vi "MakeErrorObsolete.vi"(8 "ErrorIn":errorcluster caption="Error In(no Error)", 10 "ErrorCode":i32, 11 "ReferenceIn":refnum<class "ErrorDefinitionSQLite.lvclass"> caption="Reference In") -> (0 "ErrorOut":errorcluster caption="Error Out", 3 "ReferenceOut":refnum<class "ErrorDefinitionSQLite.lvclass"> caption="Reference Out")   [LabVIEW 2018, in "ErrorDefinitionSQLite.lvclass"]
uses:
  ErrorDefinitionSQLite.lvclass
  <vilib>/drjdpowell/SQLite Library/SQL Connection/Execute SQL.vi
  <vilib>/drjdpowell/SQLite Library/SQLite.lvlib
  <vilib>/drjdpowell/SQLite Library/SQL Connection/Connection.lvclass
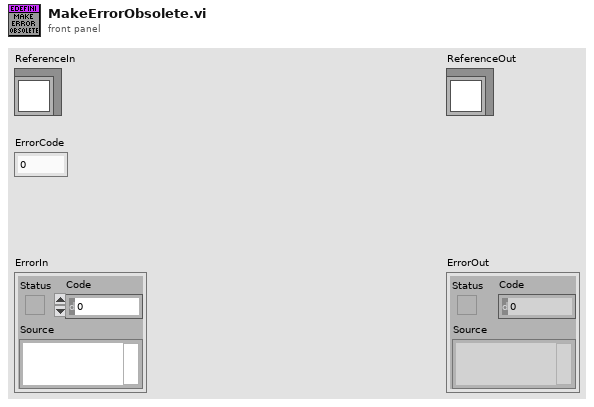
[diagram p1: front panel]
types:
  T1 = typedef "ErrorDefinitionSQLite.lvclass/ObjectAttributes.ctl" = cluster{"Path":path, "SQLiteRef":refnum<class "Connection.lvclass">, "EndOfRange":i32, "DefaultLibrarySize":i32, "StartOfRange":i32}
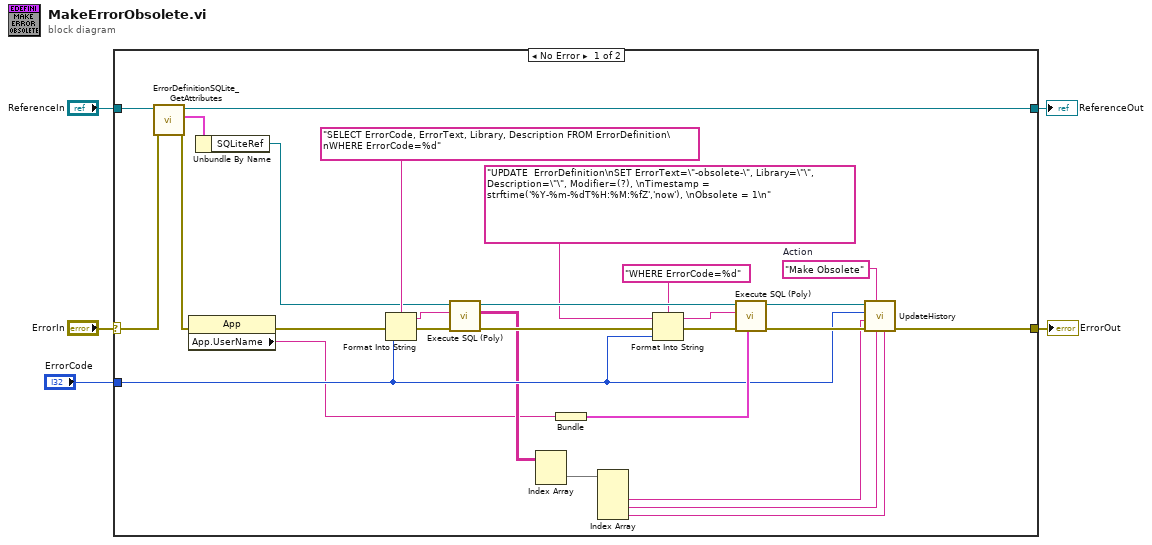
[diagram p0: block diagram]
diagram:
  n1 = case shown="No Error" "ErrorIn" {
    selector: "ErrorIn" -> [w33 w35]
    tunnel: [w6 w35] -> w4
    tunnel: [w31 w34] -> w2
    tunnel: "ReferenceIn" -> [w32 w34]
    tunnel: "ErrorCode" -> [w19 _]
    frame No Error {
      w26 = "Make Obsolete"  # Action
      n2 = call "ErrorDefinitionSQLite_GetAttributes.vi"("ErrorIn"=w33, "Reference in"=w32) -> ("ErrorOut"=w12:errorcluster, "Data"=w30:T1, "Reference out"=w31:refnum<class "ErrorDefinitionSQLite.lvclass">)  [unwired: 6 in, 1 out]
      n3 = property class="App"(error in=w12) -> (error out=w7:errorcluster, "App.UserName"=w9:string)  [unwired: 1 in, 1 out]
      n4 = Unbundle By Name(w30) -> ("SQLiteRef"=w8:refnum<class "Connection.lvclass">)
      n5 = Format Into String(format string="SELECT ErrorCode, ErrorText, Library, Description FROM ErrorDefinition\nWHERE ErrorCode=%d" ("SQL"), error in=w7, w19) -> (resulting string=w18:string, error out=w20:errorcluster)  [unwired: 1 in]
      n6 = call-poly <vilib>:"Execute SQL (Poly).vi"("error in (no error)"=w20, "SQL"=w18, "SQLite Connection in"=w8) -> ("error out"=w23:errorcluster, "Result Set"=w17:string[][], "SQLite Connection"=w22:refnum<class "Connection.lvclass">)  [unwired: 5 in, 1 out]
      n7 = Index Array(array=w17) -> (element=w16:string[])  [unwired: 2 in]
      n8 = Bundle("App.UserName"=w9) -> (w27:cluster{"App.UserName":string})  [unwired: 1 in]
      n9 = Index Array(array=w16) -> (element #2=w15:string, element #3=w14:string, element #4=w13:string)  [unwired: 4 in, 1 out]
      n10 = Format Into String(format string="WHERE ErrorCode=%d" ("SQL"), initial string="UPDATE  ErrorDefinition\nSET ErrorText=\"-obsolete-\", Library=\"\", Description=\"\", Modifier=(?), \nTimestamp = strftime('%Y-%m-%dT%H:%M:%fZ','now'), \nObsolete = 1\n" ("SQL"), error in=w23, w19) -> (resulting string=w28:string, error out=w29:errorcluster)
      n11 = call-poly <vilib>:"Execute SQL (Poly).vi"("Parameter(s)"=w27, "error in (no error)"=w29, "SQL"=w28, "SQLite Connection in"=w22) -> ("error out"=w24:errorcluster, "SQLite Connection"=w25:refnum<class "Connection.lvclass">)  [unwired: 4 in, 2 out]
      n12 = call "UpdateHistory.vi"("Description"=w13, "Library"=w14, "Action"=w26, "error in (no error)"=w24, "ErrorText"=w15, "ErrorCode"=w19, "Connection in"=w25) -> ("error out"=w6:errorcluster)  [unwired: 3 in, 1 out]
    }
    frame Error {
    }
  }
  "ErrorOut" <- w4
  "ReferenceOut" <- w2
